vi "n set io bit.vi"(8 "error in (no error)":errorcluster, 10 "mask1":u16, 11 "n":u16) -> (0 "error out":errorcluster)   [LabVIEW 2015, in "SCANalone4x64.lvlib"]
doc: "__declspec(dllimport) void __stdcall n_set_io_bit(unsigned short n, unsigned short mask1);"
uses:
  <userlib>/SCANalone4x64/SCANalone4x64.lvlib
  <userlib>/SCANalone4x64/SCANalone4x64.dll
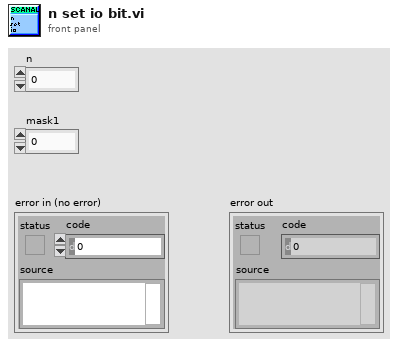
[diagram p1: front panel]
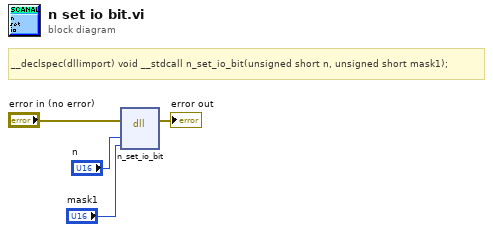
[diagram p0: block diagram]
diagram:
  # "__declspec(dllimport) void __stdcall n_set_io_bit(unsigned short n, unsigned short mask1);"
  n1 = dll-call lib="C:/Program Files/National Instruments/LabVIEW 2015/user.lib/SCANalone4x64/SCANalone4x64.*" fn="n_set_io_bit"(error in="error in (no error)", "n"="n", "mask1"="mask1") -> (error out=→"error out":errorcluster)  [unwired: 5 in, 1 out]
